vi "Set Port Status_UI Actor.vi"(6 "Byte 0":string(combo), 8 "error in (no error)":errorcluster, 9 "Byte 1":string(combo), 10 "CH":i32, 11 "UI Actor in":refnum<class "UI Actor.lvclass">) -> (0 "error out":errorcluster, 3 "UI Actor out":refnum<class "UI Actor.lvclass">)   [LabVIEW 2020, in "UI Actor.lvlib" / "UI Actor.lvclass"]
uses:
  UI Actor.lvclass
  UI Actor.lvclass/UI Actor.ctl
  Abstract/Serial Device/Serial Device.lvclass
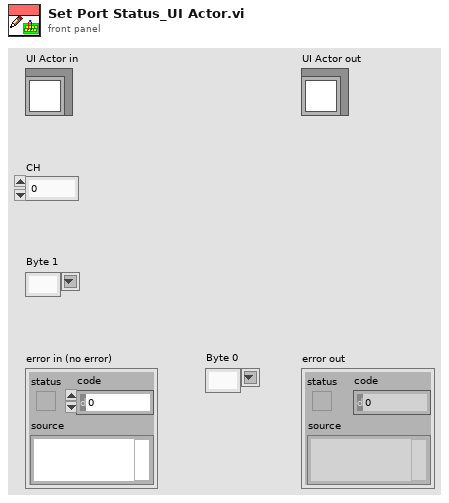
[diagram p1: front panel]
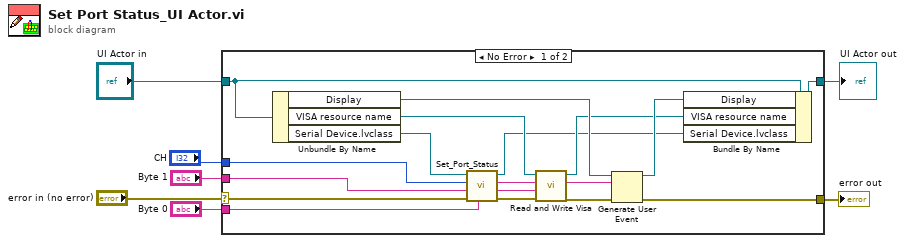
[diagram p0: block diagram]
diagram:
  n1 = case shown="No Error" "error in (no error)" {
    selector: "error in (no error)" -> [w14 w27]
    tunnel: [w9 w27] -> w6
    tunnel: [w8 w26] -> w4
    tunnel: "UI Actor in" -> [w10 w26]
    tunnel: "CH" -> [w11 _]
    tunnel: "Byte 0" -> [w13 _]
    tunnel: "Byte 1" -> [w12 _]
    frame No Error {
      n2 = Unbundle By Name(w10) -> ("Display"=w25:refnum<user-event>, "VISA resource name"=w24:refnum<visa-resource-name>, "Serial Device.lvclass"=w19:refnum<class "Serial Device.lvclass">)
      n3 = call-dynamic "Set_Port_Status.vi"("Byte 0"=w13, "error in (no error)"=w14, "Byte 1"=w12, "CH"=w11, "Serial Device in"=w19) -> ("error out"=w17:errorcluster, "Expected Response"=w16:string, "Command to Send"=w15:string, "Serial Device out"=w18:refnum<class "Serial Device.lvclass">)  [unwired: 3 in]
      n4 = call "Read and Write Visa.vi"("error in (no error)"=w17, "Expected Response"=w16, "Command to Send"=w15, "VISA Refnum in"=w24) -> ("error out"=w23:errorcluster, "Expected Response out"=w22:string, "VISA Refnum out"=w20:refnum<visa-resource-name>)  [unwired: 5 in]
      n5 = Generate User Event(user event=w25, event data cluster=w22, error in=w23) -> (user event out=w21:refnum<user-event>, error out=w9:errorcluster)  [unwired: 1 in]
      n6 = Bundle By Name(cluster=w10, "Display"=w21, "VISA resource name"=w20, "Serial Device.lvclass"=w18) -> (w8:refnum<class "UI Actor.lvclass">)
    }
    frame Error {
    }
  }
  "error out" <- w6
  "UI Actor out" <- w4
